vi "PH_Get6PInformation.get Beckhoff Configuration.vi"(5 "error in (no error)":errorcluster) -> (19 "error out":errorcluster)   [LabVIEW 2014, in "PH_Get6PInformation.lvlib"]
doc: "This VI is forseen to to check the axis type depending settings of Beckhoff StepMot axes."
uses:
  PH_Get6PInformation.lvlib
  PH_Stepmotor_BaseClass/PH_Stepmotor_BaseClass.Motor Type.ctl
  non_GPL/instr.lib/Beckhoff/Specials/Step Motor Klemmen/Beckhoff.Step Motor - Motor Configuration.ctl
  non_GPL/instr.lib/Beckhoff/Read and Write Register/Step Motor Klemmen/Beckhoff.Step Motor - Feature Register 1.ctl
  non_GPL/instr.lib/Beckhoff/Read and Write Register/Step Motor Klemmen/Beckhoff.Step Motor - Feature Register 2.ctl
  PH_Stepmotor_BaseClass/PH_Stepmotor_BaseClass.lvlib
  PH_Beckhoff_StepMot/PH_Beckhoff_StepMot.lvlib
  non_GPL/instr.lib/Beckhoff/Beckhoff - Driver np.lvlib
panel:
  out "Step Motor Configuration":T1
  in  "Delete":bool
  in  "Motor Type":T4
  # "PCS"
  # "3.40"
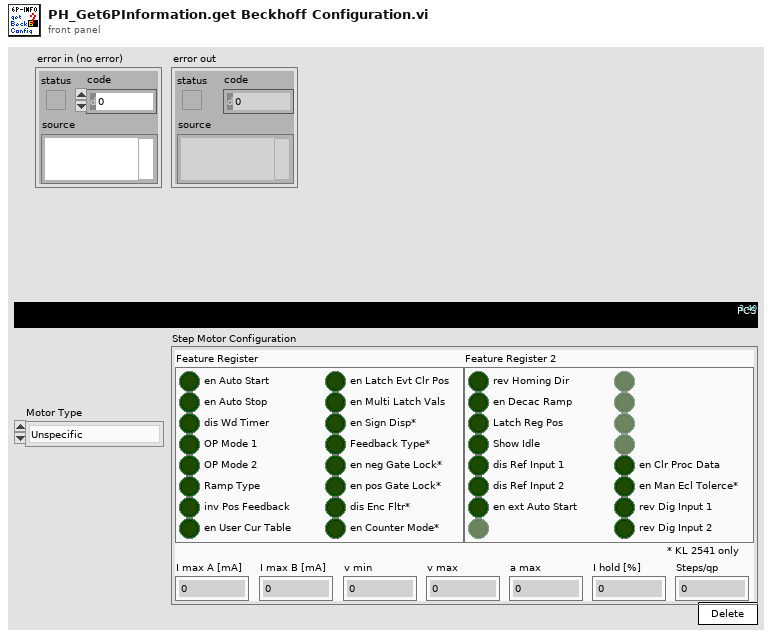
[diagram p1: front panel]
types:
  T1 = typedef "Beckhoff - Driver np.lvlib/Beckhoff.Step Motor - Motor Configuration.ctl" = cluster{"Feature Register":T2, "I max A [mA]":dbl, "I max B [mA]":dbl, "v min":u32, "v max":u32, "a max":u32, "I hold [%]":u32, "Steps/qp":u32, "Feature Register 2":T3}
  T2 = typedef "Beckhoff - Driver np.lvlib/Beckhoff.Step Motor - Feature Register 1.ctl" = cluster{"en Auto Start":bool, "en Auto Stop":bool, "dis Wd Timer":bool, "OP Mode 1":bool, "OP Mode 2":bool, "Ramp Type":bool, "inv Pos Feedback":bool, "en User Cur Table":bool, "en Latch Evt Clr Pos":bool, "en Multi Latch Vals":bool, "en Sign Disp*":bool, "Feedback Type*":bool, "en neg Gate Lock*":bool, "en pos Gate Lock*":bool, "dis Enc Fltr*":bool, "en Counter Mode*":bool}
  T3 = typedef "Beckhoff - Driver np.lvlib/Beckhoff.Step Motor - Feature Register 2.ctl" = cluster{"rev Homing Dir":bool, "en Decac Ramp":bool, "Latch Reg Pos":bool, "Show Idle":bool, "dis Ref Input 1":bool, "dis Ref Input 2":bool, "en ext Auto Start":bool, "N/A":bool, "N/A":bool, "N/A":bool, "N/A":bool, "N/A":bool, "en Clr Proc Data":bool, "en Man Ecl Tolerce*":bool, "rev Dig Input 1":bool, "rev Dig Input 2":bool}
  T4 = typedef "PH_Stepmotor_BaseClass.lvlib/PH_Stepmotor_BaseClass.Motor Type.ctl" = enum16{"Unspecific", "OWIS 49.120.2633", "OWIS 49.060.1033", "OWIS 43.040.2558", "Diamond Motion 2200 series", "OWIS 49.120.266B.MV6", "Calorimeter", "Linear Stage 1", "MICOS VT-80", "MICOS VT-80 S", "Standa Rotstage nt0.95A", "PUF RA 320.200", "PUF RA 800.200", "PUF RA 800.400", "PUF RA 400.50", "1324.nn.800.50", "1324.n9c.800.50", "1324.nn.320.200", "1324.nn.400.200", "1324.nn.800.200", "1324.nn.400.50", "1324.8c9c.800.50", "1324.8c9c.400.200"}
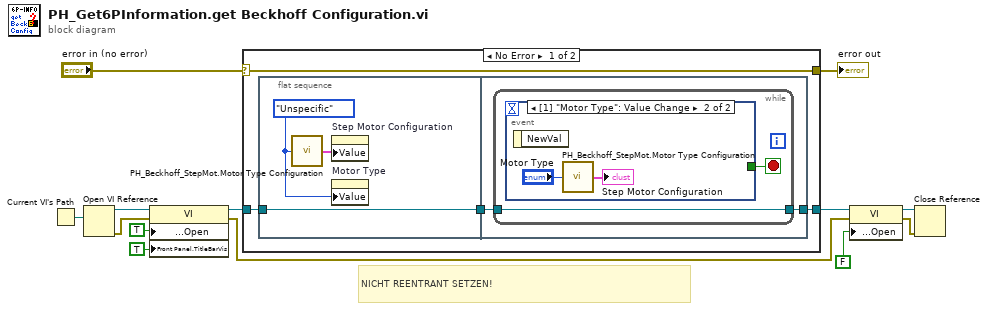
[diagram p0: block diagram]
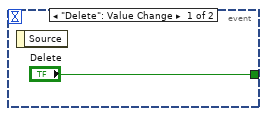
[diagram p2: hidden frame]
diagram:
  # "NICHT REENTRANT SETZEN!"
  n1 = Current VI's Path() -> (path=w11:path)
  n2 = Open VI Reference(vi path=w11) -> (vi reference=w1:refnum<vi>, error out=w5:errorcluster)  [unwired: 5 in]
  n3 = property class="VI"(reference=w1, error in=w5, "Front Panel Window:Open"=TRUE, "Front Panel.TitleBarVis"=TRUE ("Front Panel Window:Title Bar Visible")) -> (reference out=w9:refnum<vi>, error out=w4:errorcluster)
  n4 = case shown="No Error" "error in (no error)" {
    selector: "error in (no error)" -> [w17 w29]
    tunnel: [w17 w29] -> w13
    tunnel: w9 -> [w16 w28]
    tunnel: [w15 w28] -> w7
    frame No Error {
      n5 = flat-sequence {
        tunnel: w16 -> [w20]
        tunnel: [w20] -> w14
        tunnel: [w21] -> w15
        tunnel: w14 -> [w22]
        frame #0 {
          w19 = PH_Stepmotor_BaseClass.Motor_Type."Unspecific" ("Motor Type")
          n6 = call "PH_Beckhoff_StepMot.Motor Type Configuration.vi"("Motor Type"=w19) -> ("Step Motor Configuration"=w18:T1)
          n7 = property on="Step Motor Configuration" class="Clust (strict)"("Value"=w18) -> ()  [unwired: 2 in, 2 out]
          n8 = property on="Motor Type" class="Enum (strict)"("Value"=w19) -> ()  [unwired: 2 in, 2 out]
        }
        frame #1 {
          n9 = while {
            tunnel: w22 -> [w24]
            tunnel: [w24] -> w21
            stop <- w23 stop-if-true
            n10 = event shown="[1] \"Motor Type\": Value Change" {
              selector: _ -> [_ _]
              dyn-events: _ -> [_ _]
              timeout: _ -> [_ _]
              tunnel: ["Delete" _] -> w23
              event "Delete": Value Change {
                n11 = event-data() -> ()  [unwired: 1 in, 1 out]
              }
              event Value Change {
                n12 = event-data() -> ()  [unwired: 1 in, 1 out]
                n13 = call "PH_Beckhoff_StepMot.Motor Type Configuration.vi"("Motor Type"="Motor Type") -> ("Step Motor Configuration"=→"Step Motor Configuration":T1)
              }
            }
          }
        }
      }
    }
    frame Error {
    }
  }
  "error out" <- w13
  n14 = property class="VI"(reference=w7, error in=w4, "Front Panel Window:Open"=FALSE) -> (reference out=w6:refnum<vi>, error out=w3:errorcluster)
  n15 = Close Reference(reference=w6, error in (no error)=w3) -> ()  [unwired: 1 out]
